vi "Blank VI 01.vi"() -> ()   [LabVIEW 2016]
panel:
  in  "Exit":bool
  out "Numeric":i32
  in  "Calling VI Ref":refnum<vi>
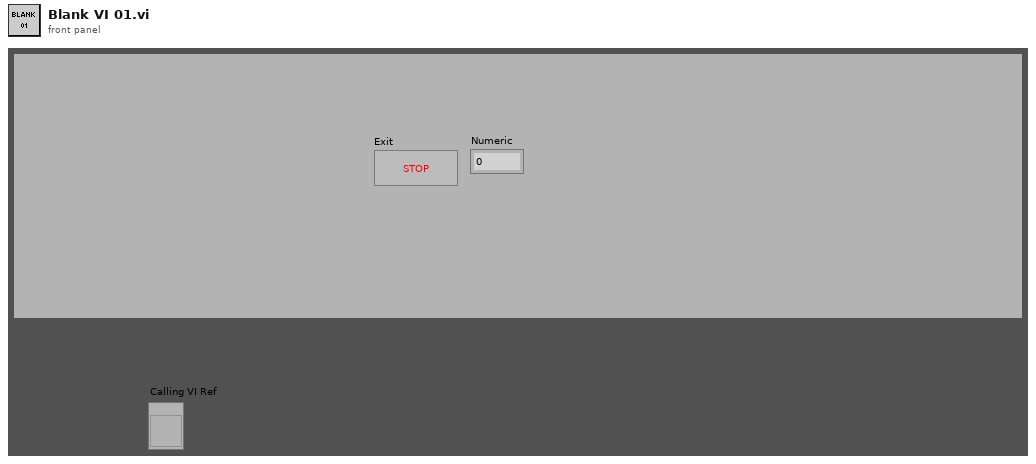
[diagram p1: front panel]
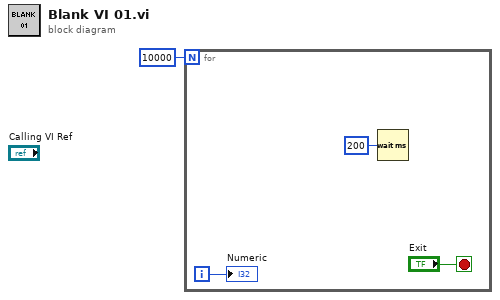
[diagram p0: block diagram]
diagram:
  n1 = for {
    N: 10000 -> [_]
    i -> [w3]
    stop <- "Exit" stop-if-true
    n2 = Wait (ms)(milliseconds to wait=u32 200) -> ()  [unwired: 1 out]
    "Numeric" <- w3
  }
